vi "usrp get gpio attr.vi"(6 "attr_out":u32, 7 "mboard":u64, 8 "error in (no error)":errorcluster, 9 "attr":string, 10 "bank":string, 11 "h":u64) -> (0 "error out":errorcluster, 3 "function return":u32(ring), 4 "attr_out out":u32)   [LabVIEW 2023, in "uhd.lvlib"]
doc: "UHD_API uhd_error uhd_usrp_get_gpio_attr(uhd_usrp_handle h,\n const char* bank,\n const char* attr,\n size_t mboard,\n uint32_t* attr_out);"
uses:
  <userlib>/uhd/uhd.lvlib
  <userlib>/uhd/uhd.dll
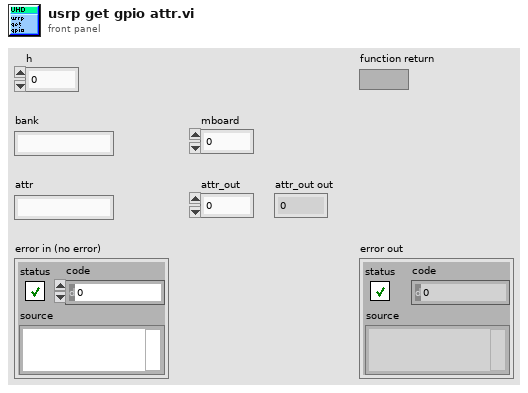
[diagram p1: front panel]
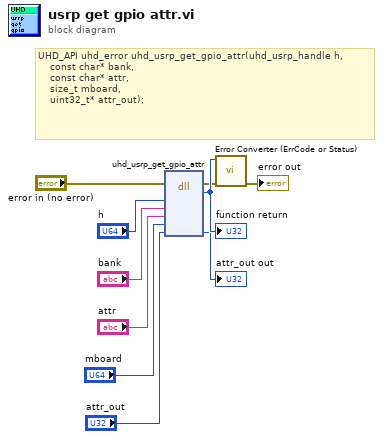
[diagram p0: block diagram]
diagram:
  # "UHD_API uhd_error uhd_usrp_get_gpio_attr(uhd_usrp_handle h,\n    const char* bank,\n    const char* attr,\n    size_t mboard,\n    uint32_t* attr_out);"
  n1 = dll-call lib="C:/Program Files/National Instruments/LabVIEW 2023/user.lib/uhd/uhd.*" fn="uhd_usrp_get_gpio_attr"(error in="error in (no error)", "h"="h", "bank"="bank", "attr"="attr", "mboard"="mboard", "attr_out"="attr_out") -> (error out=w2:errorcluster, w10:u32, "attr_out"=→"attr_out out":u32)  [unwired: 6 in, 1 out]
  "function return" <- w10
  n2 = call <userlib>:"Error Converter (ErrCode or Status).vi"("error in (no error)"=w2, "error code"=w10) -> ("error out"=→"error out":errorcluster)  [unwired: 9 in]
